vi "TurnSmooth.vi"(5 "Min Power":dbl, 6 "First Time?":bool, 7 "Target Range":dbl, 8 "Current Position":dbl, 9 "Target Position":dbl, 10 "Slow Range":dbl, 11 "Motor Power In":dbl) -> (0 "Done":bool, 2 "Right Motor Power":dbl, 3 "Left Motor Power":dbl)   [LabVIEW 2016]
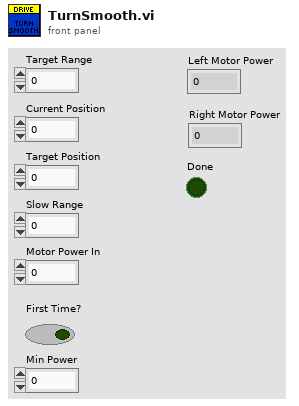
[diagram p1: front panel]
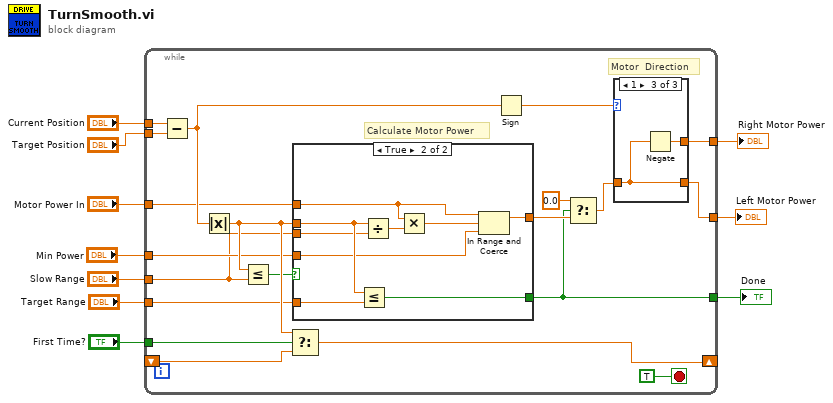
[diagram p0: block diagram]
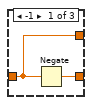
[diagram p2: hidden frame]
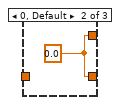
[diagram p3: hidden frame]
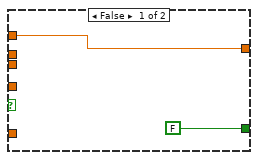
[diagram p4: hidden frame]
diagram:
  n1 = while {
    shift-right: [w28] -> _
    shift-left: _ -> [w29]
    tunnel: [w13] -> w10
    tunnel: [w23] -> w9
    tunnel: [w22] -> w8
    tunnel: "Current Position" -> [w21]
    tunnel: "Target Position" -> [w20]
    tunnel: "Motor Power In" -> [w19]
    tunnel: "Min Power" -> [w18]
    tunnel: "Slow Range" -> [w11]
    tunnel: "Target Range" -> [w17]
    tunnel: "First Time?" -> [w16]
    stop <- TRUE stop-if-true
    # "Motor  Direction"
    # "Calculate Motor Power"
    n2 = Subtract(x=w21, y=w20) -> (x-y=w25:dbl)
    n3 = Absolute Value(x=w25) -> (abs(x)=w27:dbl)
    n4 = Less Or Equal?(x=w27, y=w11) -> (x <= y?=w26:bool)
    n5 = Select(t=w27, s=w16, f=w29) -> (s? t:f=w28:dbl)
    n6 = case shown="True" w26 {
      tunnel: w27 -> [_ w43]
      tunnel: w17 -> [_ w44]
      tunnel: [FALSE w41] -> w13
      tunnel: [w36 w46] -> w15
      tunnel: w19 -> [w36 w45]
      tunnel: w18 -> [_ w42]
      tunnel: w11 -> [_ w40]
      frame False {
      }
      frame True {
        n7 = Less Or Equal?(x=w43, y=w44) -> (x <= y?=w41:bool)
        n8 = Divide(x=w43, y=w40) -> (x/y=w38:dbl)
        n9 = Multiply(x=w45, y=w38) -> (x*y=w39:dbl)
        n10 = In Range and Coerce(upper limit=w45, x=w39, lower limit=w42) -> (coerced(x)=w46:dbl)  [unwired: 1 out]
      }
    }
    n11 = Sign(1:w25) -> (0:w24:dbl)
    n12 = Select(t=0.0, s=w13, f=w15) -> (s? t:f=w14:dbl)
    n13 = case shown="1" w24 {
      tunnel: [w32 w33 w34] -> w23
      tunnel: [w31 w33 w35] -> w22
      tunnel: w14 -> [w31 _ w34]
      frame -1 {
        n14 = Negate(x=w31) -> (-x=w32:dbl)
      }
      frame 0, Default {
        w33 = 0.0
      }
      frame 1 {
        n15 = Negate(x=w34) -> (-x=w35:dbl)
      }
    }
  }
  "Left Motor Power" <- w9
  "Done" <- w10
  "Right Motor Power" <- w8
